vi "Validate Route part 2.vi"(10 "Path":T1[](array[typedef]), 11 "All Caves":T1[](array[typedef])) -> (2 "End?":bool, 3 "Invalid Path?":bool)   [LabVIEW 2019, in "Day 12.lvlib"]
uses:
  Day 12.lvlib
  Controls/Cave.ctl
  Controls/Cave Type.ctl
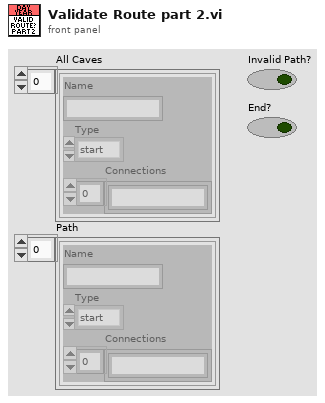
[diagram p1: front panel]
types:
  T1 = typedef "Day 12.lvlib/Cave.ctl" = cluster{"Name":string, "Type":T2, "Connections":string[]}
  T2 = typedef "Day 12.lvlib/Cave Type.ctl" = enum16{"start", "end", "small", "big"}
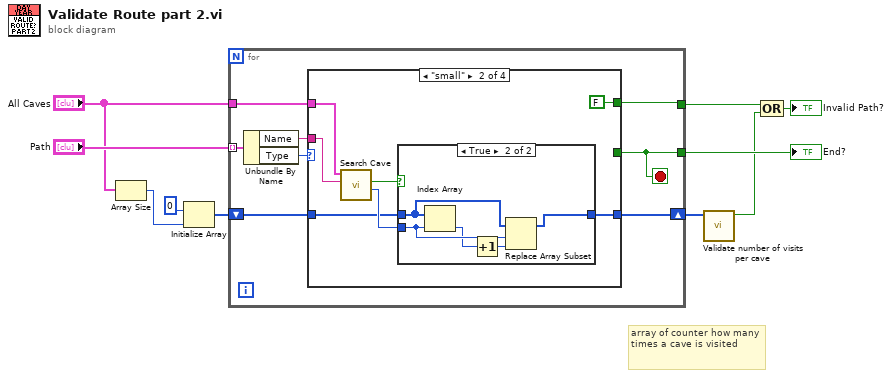
[diagram p0: block diagram]
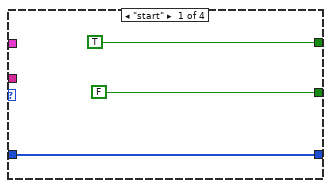
[diagram p2: hidden frame]
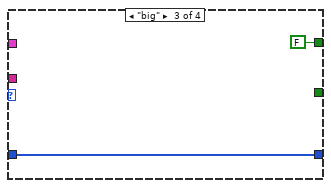
[diagram p4: hidden frame]
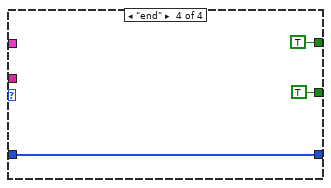
[diagram p5: hidden frame]
diagram:
  # "array of counter how many times a cave is visited"
  n1 = Array Size(array="All Caves") -> (size(s)=w7:i32)
  n2 = Initialize Array(0 ("Cave counter"), w7) -> (w6:i32[])
  n3 = for {
    tunnel: "Path" -> [w18] mode=indexing
    shift-right: [w13] -> w4
    shift-left: w6 -> [w14]
    tunnel: [w16] -> w10
    tunnel: [w15] -> w3
    tunnel: "All Caves" -> [w12]
    stop <- w16 stop-if-true
    n4 = Unbundle By Name(w18) -> ("Name"=w11:string, "Type"=w17:T2)
    n5 = case shown="\"small\"" w17 {
      tunnel: [FALSE _ _ TRUE] -> w16
      tunnel: [TRUE FALSE FALSE TRUE] -> w15
      tunnel: w14 -> [w19 w24 w36 w38]
      tunnel: [w19 w23 w36 w38] -> w13
      tunnel: w12 -> [_ w28 _ _]
      tunnel: w11 -> [_ w27 _ _]
      frame "start" {
      }
      frame "small" {
        n6 = call "Search Cave.vi"("Cave Name"=w27, "Caves"=w28) -> ("Index"=w25:i32, "Found?"=w26:bool)  [unwired: 7 in, 1 out]
        n7 = case shown="True" w26 {
          tunnel: w25 -> [_ w33]
          tunnel: w24 -> [w29 w34]
          tunnel: [w29 w30] -> w23
          frame False {
          }
          frame True {
            n8 = Index Array(array=w34, index=w33) -> (element=w32:i32)
            n9 = Increment(x=w32) -> (x+1=w31:i32)
            n10 = Replace Array Subset(array=w34, new element=w31, index=w33) -> (w30:i32[])
          }
        }
      }
      frame "big" {
      }
      frame "end" {
      }
    }
  }
  "End?" <- w10
  n11 = call "Validate number of visits per cave.vi"("Array"=w4) -> ("Invalid?"=w1:bool)  [unwired: 10 in]
  n12 = Compound Arithmetic op=OR(w3, w1) -> (→"Invalid Path?":bool)
